vi "Move Slit.vi"(7 "Mono System # (0)":T2, 8 "error in (no error)":errorcluster, 9 "Desired Slit Position":dbl[unit], 10 "Slit (Front/Axial Entrance)":T1, 11 "VISA resource name":refnum<visa-resource-name>) -> (0 "error out":errorcluster, 3 "VISA resource name out":refnum<visa-resource-name>)   [LabVIEW 2017, in "JY-SPEX-TRIAX.lvlib"]
doc: "Moves the spectrometer's slits to the specified position. Returns control after the slits are done moving.\n\nA positive number of steps opens the slits wider, while a negative makes them narrower. This command corrects for backlash automatically.\n\nOnly one stepper motor can move at a time; thus, this command waits if either other slits or the wavelength drive are being moved.\n\nThe limit to the number of steps that can be moved is the total number of possible steps for the slit."
uses:
  JY-SPEX-TRIAX.lvlib
  controls.llb/Monochromator System Number.ctl
  controls.llb/Slits.ctl
  Spectrometer Config.vi
panel:
  out "Target":dbl[unit]
  out "Steps":i32
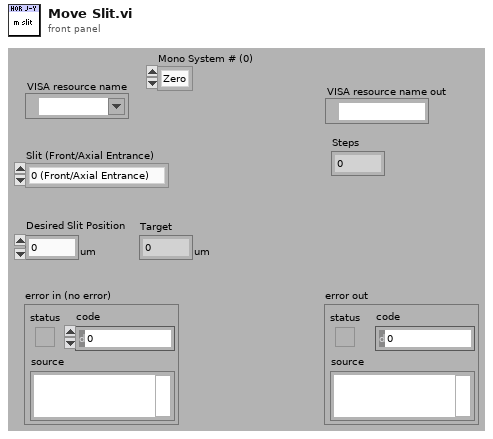
[diagram p1: front panel]
types:
  T1 = typedef "JY-SPEX-TRIAX.lvlib/Slits.ctl" = enum16{"0 (Front/Axial Entrance)", "1 (Side/Lateral Entrance)", "2 (Front/Axial Exit)", "3 (Side/Lateral Exit)"}
  T2 = typedef "JY-SPEX-TRIAX.lvlib/Monochromator System Number.ctl" = enum16{"Zero", "One"}
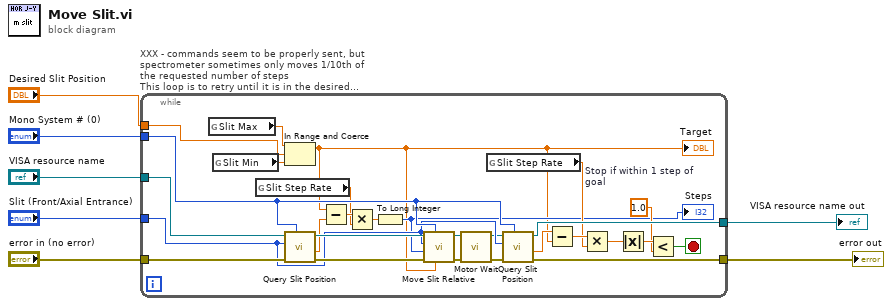
[diagram p0: block diagram]
diagram:
  n1 = while "XXX - commands seem to be properly sent, but spectrometer sometimes only moves 1/10th of the requested number of steps\nThis loop is to retry until it is in the desired position" {
    tunnel: "VISA resource name" -> [w35]
    tunnel: "error in (no error)" -> [w34]
    tunnel: "Desired Slit Position" -> [w33]
    tunnel: "Mono System # (0)" -> [w21]
    tunnel: "Slit (Front/Axial Entrance)" -> [w20]
    tunnel: [w30] -> w2
    tunnel: [w29] -> w1
    stop <- w23 stop-if-true
    w24 = 1.0  # Stop if within 1 step of goal
    n2 = global read "Spectrometer Config.vi" "Slit Max"() -> (w16:dbl[unit])
    n3 = global read "Spectrometer Config.vi" "Slit Min"() -> (w17:dbl[unit])
    n4 = global read "Spectrometer Config.vi" "Slit Step Rate"() -> (w14:dbl[unit])
    n5 = In Range and Coerce(upper limit=w16, x=w33, lower limit=w17) -> (coerced(x)=w8:dbl[unit])  [unwired: 1 out]
    "Target" <- w8
    n6 = call "Query Slit Position.vi"("Mono System # (0)"=w21, "error in (no error)"=w34, "Slit (Front/Axial Entrance)"=w20, "VISA resource name"=w35) -> ("error out"=w31:errorcluster, "Slit Position"=w19:dbl[unit], "VISA resource name out"=w32:refnum<visa-resource-name>)  [unwired: 5 out]
    n7 = Subtract(x=w8, y=w19) -> (x-y=w18:dbl[unit])
    n8 = Multiply(x=w18, y=w14) -> (x*y=w15:dbl)
    n9 = To Long Integer(number=w15) -> (32bit integer=w13:i32)
    "Steps" <- w13
    n10 = call "Move Slit Relative.vi"("Target"=w8, "Mono System # (0)"=w21, "error in (no error)"=w31, "Steps to Move"=w13, "Slit (Front/Axial Entrance)"=w20, "VISA resource name"=w32) -> ("error out"=w11:errorcluster, "VISA resource name out"=w12:refnum<visa-resource-name>)  [unwired: 4 out]
    n11 = call "Motor Wait.vi"("error in"=w11, "VISA resource name in"=w12) -> ("error out"=w9:errorcluster, "VISA resource name out"=w10:refnum<visa-resource-name>)  [unwired: 8 out]
    n12 = global read "Spectrometer Config.vi" "Slit Step Rate"() -> (w22:dbl[unit])
    n13 = call "Query Slit Position.vi"("Mono System # (0)"=w21, "error in (no error)"=w9, "Slit (Front/Axial Entrance)"=w20, "VISA resource name"=w10) -> ("error out"=w29:errorcluster, "Slit Position"=w28:dbl[unit], "VISA resource name out"=w30:refnum<visa-resource-name>)  [unwired: 5 out]
    n14 = Subtract(x=w28, y=w8) -> (x-y=w27:dbl[unit])
    n15 = Multiply(x=w27, y=w22) -> (x*y=w26:dbl)
    n16 = Absolute Value(x=w26) -> (abs(x)=w25:dbl)
    n17 = Less?(x=w25, y=w24) -> (x < y?=w23:bool)
  }
  "VISA resource name out" <- w2
  "error out" <- w1
